vi "Time_Histogram.vi"(3 "Hist array in":u16[][](array[numeric]), 4 "Max (s)":sgl=0.25 format="%#_13g", 5 "Data in":u16[](array[numeric])) -> (1 "Hist array out":u16[][](array[numeric]))   [LabVIEW 2014]
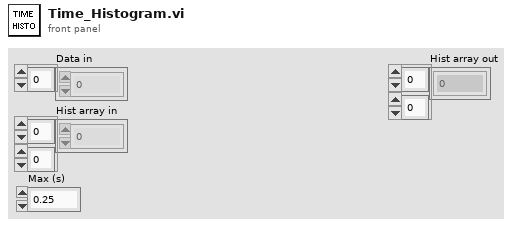
[diagram p1: front panel]
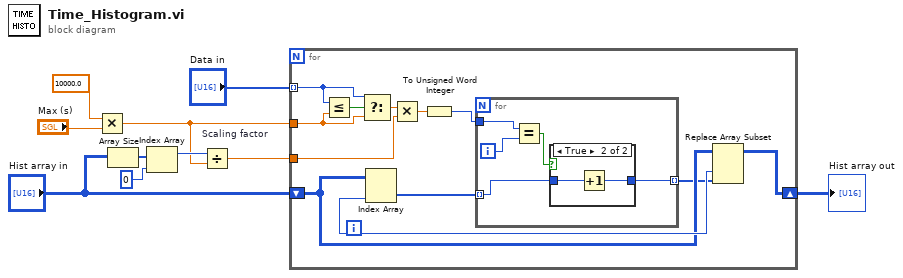
[diagram p0: block diagram]
diagram:
  n1 = Multiply(x=10000.0, y="Max (s)") -> (x*y=w1:dbl)
  n2 = Array Size(array="Hist array in") -> (size(s)=w6:i32[])
  n3 = Index Array(array=w6, index=0) -> (element=w5:i32)
  n4 = Divide "Scaling factor"(x=w5, y=w1) -> (x/y=w4:dbl)
  n5 = for {
    tunnel: "Data in" -> [w21] mode=indexing
    shift-right: [w15] -> w9
    shift-left: "Hist array in" -> [w17]
    tunnel: w1 -> [w14]
    tunnel: w4 -> [w13]
    i -> [w18]
    n6 = Less Or Equal?(x=w21, y=w14) -> (x <= y?=w22:bool)
    n7 = Select(t=w21, s=w22, f=w14) -> (s? t:f=w19:dbl)
    n8 = Index Array(array=w17, index (col)=w18) -> (element=w20:u16[])  [unwired: 1 in]
    n9 = Multiply(x=w19, y=w13) -> (x*y=w11:dbl)
    n10 = To Unsigned Word Integer(number=w11) -> (unsigned 16bit integer=w12:u16)
    n11 = for {
      tunnel: w20 -> [w27] mode=indexing
      tunnel: [w25] -> w16 mode=indexing
      tunnel: w12 -> [w24]
      i -> [w23]
      n12 = Equal?(x=w24, y=w23) -> (x = y?=w26:bool)
      n13 = case shown="True" w26 {
        tunnel: w27 -> [w28 w30]
        tunnel: [w28 w29] -> w25
        frame False {
        }
        frame True {
          n14 = Increment(x=w30) -> (x+1=w29:u16)
        }
      }
    }
    n15 = Replace Array Subset(array=w17, new element=w16, index (col)=w18) -> (w15:u16[][])  [unwired: 1 in]
  }
  "Hist array out" <- w9
